vi "Launch Devices.vi"(8 "error in":errorcluster, 11 "Controller In":refnum<class "Controller.lvclass">) -> (0 "error out":errorcluster, 3 "Controller Out":refnum<class "Controller.lvclass">)   [LabVIEW 2018, in "Controller.lvlib" / "Controller.lvclass"]
uses:
  Controller.lvclass
  Devices/Alicat/Session Based/Alicat Device.lvclass
  C:/Users/Labview/Documents/exscalabar_server/Devices/Configurable Device/Configurable Device.lvclass
  Devices/Vaisala Probe/Vaisala.lvclass
  Devices/PPT/PPT.lvclass
  Devices/TE Cooler/TE Cooler.lvclass
  Devices/Meerstetter TEC/Meerstetter TEC.lvclass
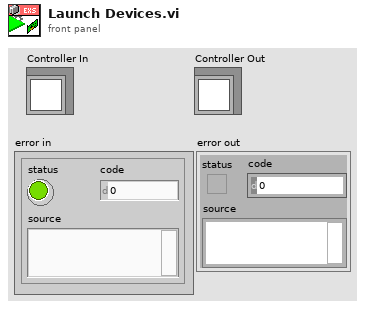
[diagram p1: front panel]
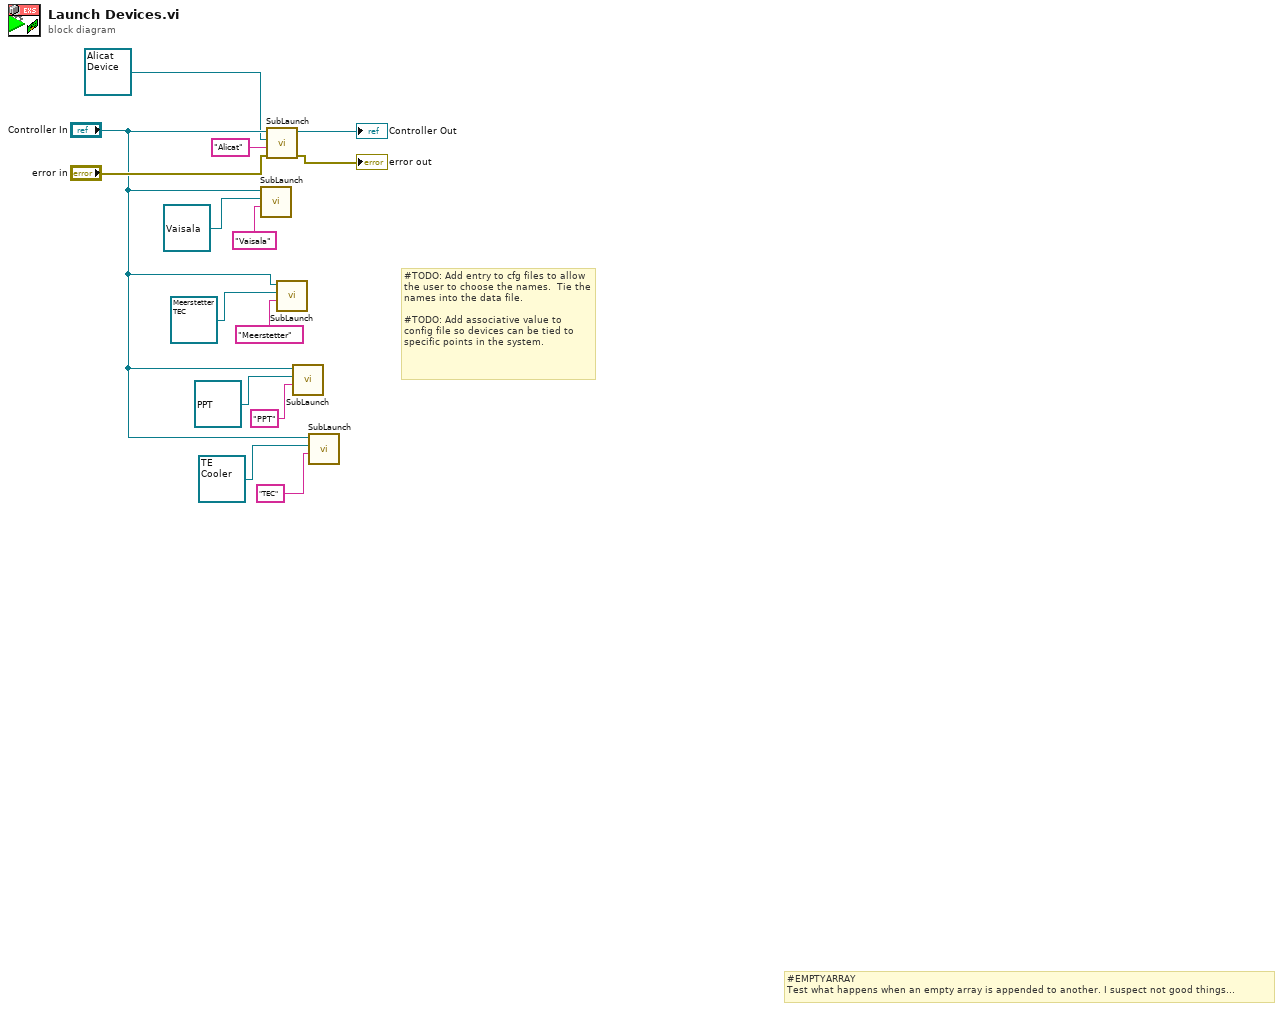
[diagram p0: block diagram]
diagram:
  # "#EMPTYARRAY\nTest what happens when an empty array is appended to another. I suspect not good things..."
  # "#TODO: Add entry to cfg files to allow the user to choose the names.  Tie the names into the data file.\n\n#TODO: Add associative value to config file so devices can be tied to specific points in the system."
  n1 = call "SubLaunch.vi"("ID"="Vaisala", "DeviceObj"=refnum<class "Vaisala.lvclass"> refnum ("Vaisala Library.lvlib:Vaisala"), "Controller in"="Controller In") -> ()  [unwired: 7 in, 2 out]
  n2 = call "SubLaunch.vi"("error in (no error)"="error in", "ID"="Alicat", "DeviceObj"=refnum<class "Alicat Device.lvclass"> refnum ("Alicat Lib.lvlib:Alicat Device"), "Controller in"="Controller In") -> ("error out"=→"error out":errorcluster, "Controller out"=→"Controller Out":refnum<class "Controller.lvclass">)  [unwired: 6 in]
  n3 = call "SubLaunch.vi"("ID"="Meerstetter", "DeviceObj"=refnum<class "Meerstetter TEC.lvclass"> refnum ("Meerstetter Lib.lvlib:TEC 1090"), "Controller in"="Controller In") -> ()  [unwired: 7 in, 2 out]
  n4 = call "SubLaunch.vi"("ID"="PPT", "DeviceObj"=refnum<class "PPT.lvclass"> refnum ("PPT Library.lvlib:PPT"), "Controller in"="Controller In") -> ()  [unwired: 7 in, 2 out]
  n5 = call "SubLaunch.vi"("ID"="TEC", "DeviceObj"=refnum<class "TE Cooler.lvclass"> refnum ("TE Cooler.lvlib:TE Tech"), "Controller in"="Controller In") -> ()  [unwired: 7 in, 2 out]
